vi "UDP发送测试.vi"(0 "发送数据":u16[](array[numeric]) format="%x", 1 "数据区字长":u16 format="%x", 2 "报文类型":u16 format="%x", 3 "发送方标识":u16 format="%x") -> ()   [LabVIEW 2010]
panel:
  out "索引号":u16 format="%x"
  in  "发送数据 2":u16[](array[numeric]) format="%x"
  in  "校验码":u16 format="%x"
  in  "控制板端口":u16
  in  "本机端口":u16
  in  "控制板IP":string
  out "字符串":string
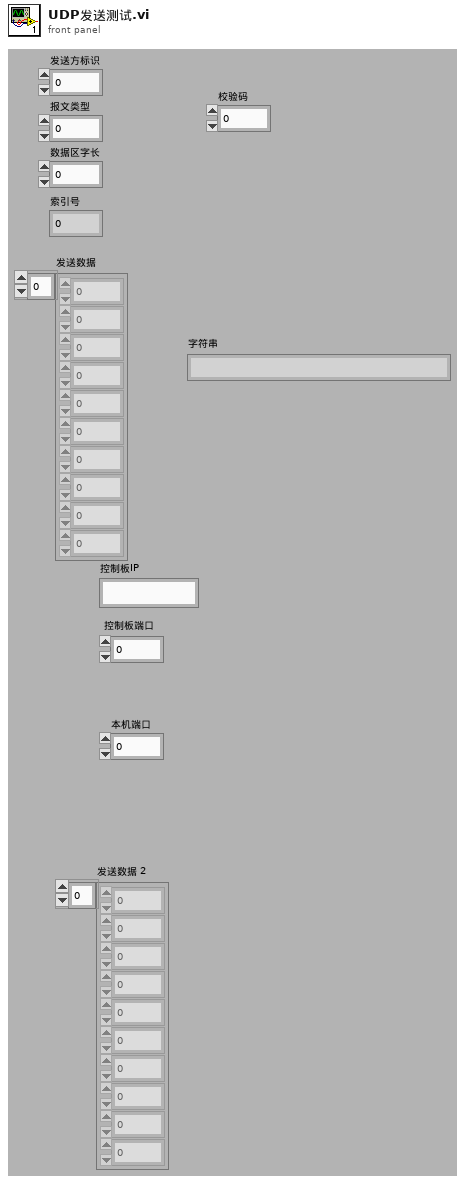
[diagram p1: front panel]
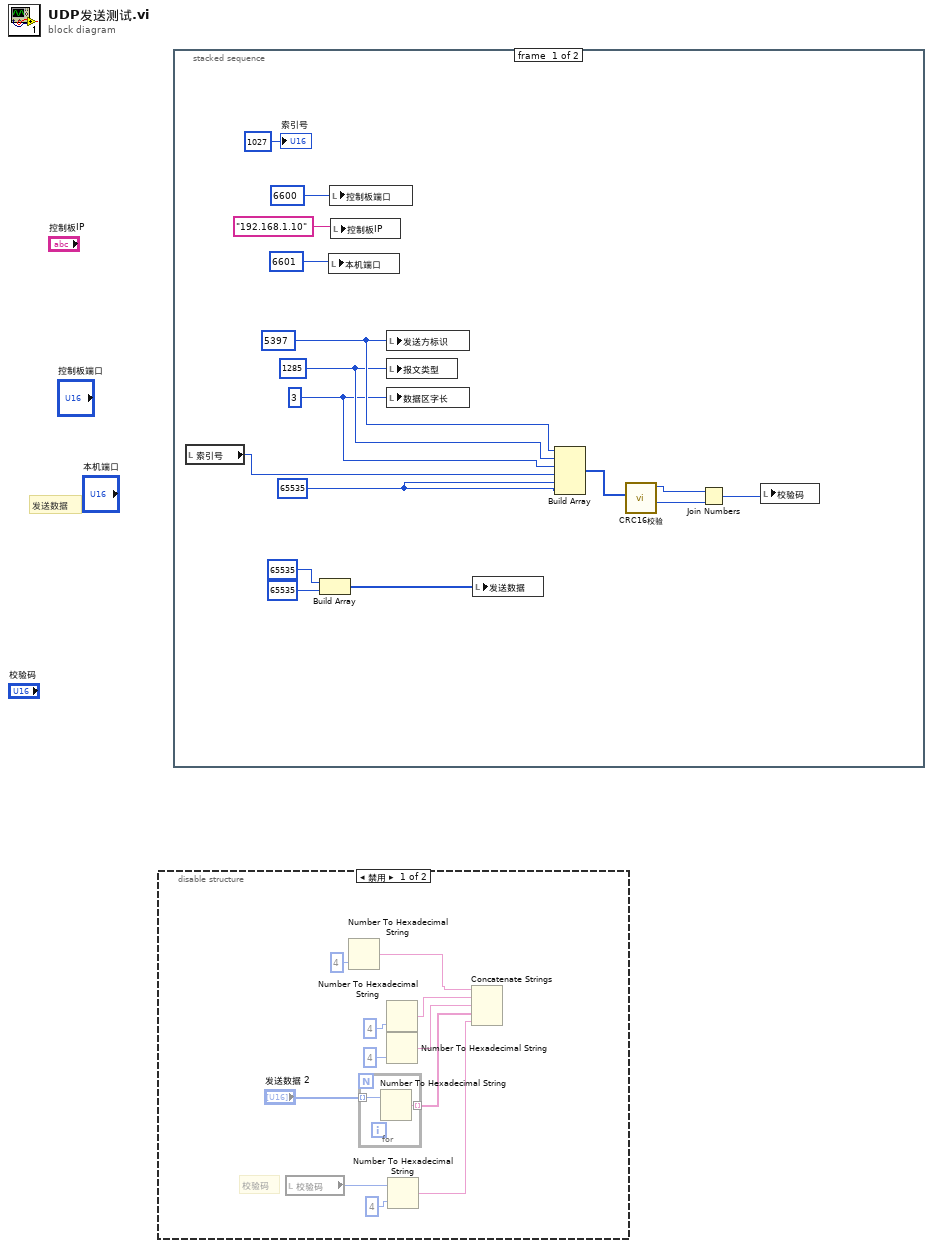
[diagram p0: block diagram]
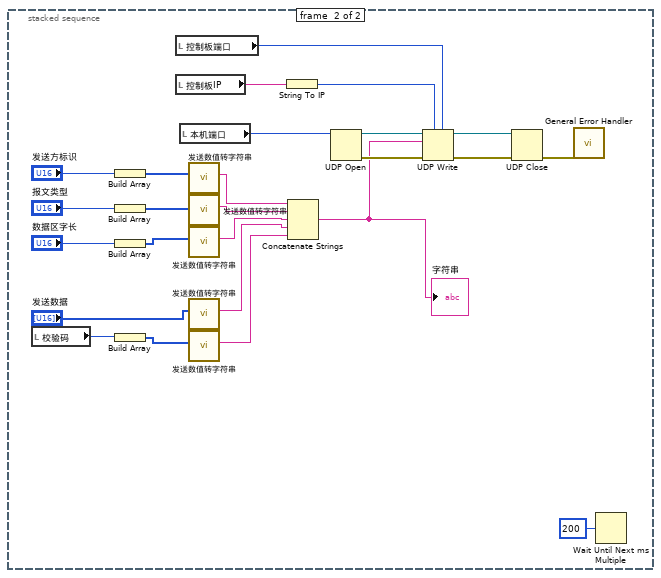
[diagram p3: hidden frame]
diagram:
  # "发送数据"
  n1 = disable-structure shown="禁用" {
    frame Disabled {
      # "校验码"
      n2 = local read "校验码"() -> (w14:u16)
      n3 = Number To Hexadecimal String(1:i16 4 ("宽度(-)")) -> (0:w13:string, 2:w12:i32)
      n4 = for {
        tunnel: "发送数据 2" -> [w16] mode=indexing
        tunnel: [w15] -> w2 mode=indexing
        n5 = Number To Hexadecimal String(2:w16) -> (0:w15:string)  [unwired: 1 in]
      }
      n6 = Number To Hexadecimal String(1:i16 4 ("宽度(-)")) -> (0:w4:string, 2:w6:i32)
      n7 = Number To Hexadecimal String(1:i16 4 ("宽度(-)")) -> (0:w3:string, 2:w5:i32)
      n8 = Number To Hexadecimal String(1:i16 4 ("宽度(-)"), 2:w14) -> (0:w1:string)
      n9 = Concatenate Strings(w13, w4, w3, w2, w1) -> ()  [unwired: 1 out]
    }
    frame Enabled {
    }
  }
  n10 = stacked-sequence {
    frame #0 {
      w17 = u16 65535 ("数据区字长")
      w19 = u16 3 ("数据区字长")
      w20 = u16 1285 ("报文类型")
      w21 = u16 5397 ("发送方标识")
      n11 = local read "索引号"() -> (w18:u16)
      n12 = Build Array(u16 65535 ("发送数据"), u16 65535 ("发送数据")) -> (w28:u16[])
      n13 = local write "本机端口"(u16 6601 ("本机端口")) -> ()
      n14 = local write "控制板端口"(u16 6600 ("控制板端口")) -> ()
      n15 = local write "控制板IP"("192.168.1.10" ("控制板IP")) -> ()
      n16 = local write "发送方标识"(w21) -> ()
      n17 = local write "报文类型"(w20) -> ()
      n18 = local write "数据区字长"(w19) -> ()
      n19 = local write "发送数据"(w28) -> ()
      n20 = Build Array(w21, w20, w19, w18, w17, w17) -> (w26:u16[])
      n21 = call "CRC16校验.vi"("输入数据_U16"=w26) -> ("低字节"=w22:u8, "高字节"=w23:u8)  [unwired: 9 in]
      n22 = Join Numbers(hi=w23, lo=w22) -> ((hi.lo)=w25:u16)
      n23 = local write "校验码"(w25) -> ()
      "索引号" <- u16 1027 ("索引号")
    }
    frame #1 {
      n24 = local read "校验码"() -> (w44:u16)
      n25 = Build Array("发送方标识") -> (w43:u16[])
      n26 = Build Array("报文类型") -> (w42:u16[])
      n27 = Build Array("数据区字长") -> (w41:u16[])
      n28 = Build Array(w44) -> (w39:u16[])
      n29 = local read "控制板端口"() -> (w49:u16)
      n30 = local read "控制板IP"() -> (w50:string)
      n31 = local read "本机端口"() -> (w48:u16)
      n32 = call "发送数值转字符串.vi"("输入数据_U16"=w43) -> ("字符串"=w38:string)  [unwired: 10 in]
      n33 = call "发送数值转字符串.vi"("输入数据_U16"=w42) -> ("字符串"=w37:string)  [unwired: 10 in]
      n34 = call "发送数值转字符串.vi"("输入数据_U16"=w41) -> ("字符串"=w36:string)  [unwired: 10 in]
      n35 = call "发送数值转字符串.vi"("输入数据_U16"="发送数据") -> ("字符串"=w35:string)  [unwired: 10 in]
      n36 = call "发送数值转字符串.vi"("输入数据_U16"=w39) -> ("字符串"=w34:string)  [unwired: 10 in]
      n37 = String To IP(1:w50) -> (0:w57:u32)
      n38 = Concatenate Strings(w38, w37, w36, w35, w34) -> (w33:string)
      "字符串" <- w33
      n39 = UDP Open(11:w48) -> (port=w52:refnum<k16>, 0:w53:errorcluster)  [unwired: 4 in, 1 out]
      n40 = UDP Write(address=w57, port or service name=w49, connection ID=w52, data in=w33, 8:w53) -> (error out=w56:errorcluster, 3:w55:refnum<k16>)  [unwired: 1 in]
      n41 = UDP Close(connection ID=w55, 8:w56) -> (error out=w54:errorcluster)  [unwired: 1 out]
      n42 = call <vilib>:"General Error Handler.vi"("error in (no error)"=w54) -> ()  [unwired: 10 in, 5 out]
      n43 = Wait Until Next ms Multiple(millisecond multiple=u32 200 ("毫秒倍数")) -> ()  [unwired: 1 out]
    }
  }
